vi "OTP - Encode.vi"(10 "Key (Private)":string, 11 "message (Private)":string) -> (3 "ciphertext (Public)":string)   [LabVIEW 2013]
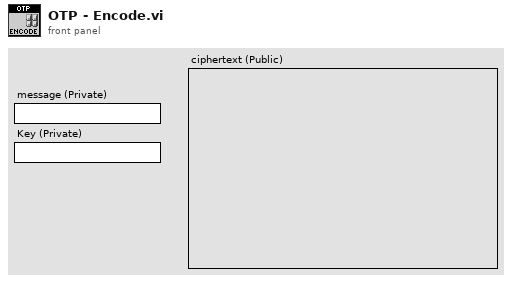
[diagram p1: front panel]
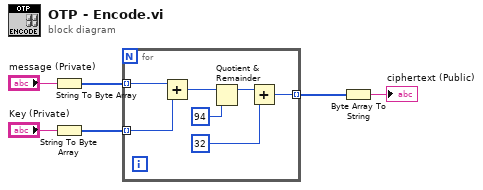
[diagram p0: block diagram]
diagram:
  n1 = String To Byte Array(string="message (Private)") -> (unsigned byte array=w2:u8[])
  n2 = String To Byte Array(string="Key (Private)") -> (unsigned byte array=w1:u8[])
  n3 = for {
    tunnel: w2 -> [w13] mode=indexing
    tunnel: [w10] -> w3 mode=indexing
    tunnel: w1 -> [w7] mode=indexing
    n4 = Add(x=w13, y=w7) -> (x+y=w12:u8)
    n5 = Quotient & Remainder(x=w12, y=u8 94) -> (x-y*floor(x/y)=w8:u8)  [unwired: 1 out]
    n6 = Add(x=w8, y=u8 32) -> (x+y=w10:u8)
  }
  n7 = Byte Array To String(unsigned byte array=w3) -> (string=→"ciphertext (Public)":string)
